vi "Read Connection Showing.vi"(8 "error in (no error)":errorcluster, 11 "Server UI in":refnum<class "Server UI.lvclass">) -> (0 "error out":errorcluster, 2 "Connection Showing":bool, 3 "Server UI out":refnum<class "Server UI.lvclass">)   [LabVIEW 2013, in "Server UI.lvlib" / "Server UI.lvclass"]
uses:
  Server UI.lvclass
  Server UI.lvclass/Server UI.ctl
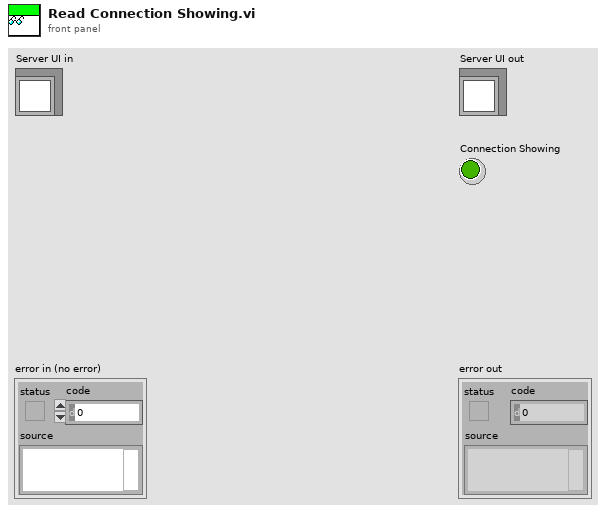
[diagram p1: front panel]
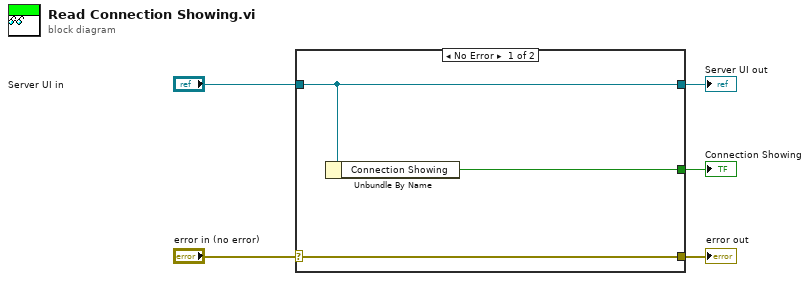
[diagram p0: block diagram]
diagram:
  n1 = case shown="No Error" "error in (no error)" {
    selector: "error in (no error)" -> [w8 w9]
    tunnel: [w8 w9] -> w4
    tunnel: [w7 w10] -> w2
    tunnel: "Server UI in" -> [w7 w10]
    tunnel: [w6 _] -> w1
    frame No Error {
      n2 = Unbundle By Name(w7) -> ("Connection Showing"=w6:bool)
    }
    frame Error {
    }
  }
  "error out" <- w4
  "Server UI out" <- w2
  "Connection Showing" <- w1
